vi "Begin.vi"() -> (0 "camera error out":errorcluster)   [LabVIEW 2013]
doc: "Called before other user functions, this VI is expected to open initial I/O refnums, load in file data, and do all program initialization. Notice that the <B>error out</B> terminal is simply used for data flow. Wiring it to other structures or subVIs ensures that this VI runs first."
uses:
  <vilib>/Rock Robotics/WPI/Encoder/WPI_EncoderType.ctl
  <vilib>/Rock Robotics/WPI/SafetyOutput/WPI_SafetyOutputConfigMenu.ctl
  <vilib>/Rock Robotics/WPI/DriverStation/WPI_DriverStationRobotMode2.ctl
  <vilib>/Rock Robotics/WPI/Joystick/WPI_JoystickDeviceEnum.ctl
  <vilib>/Rock Robotics/SystemInterfaces/DIO/FPGA_DIOPWMChannel.ctl
  <vilib>/Rock Robotics/WPI/Solenoid/WPI_SolenoidChannel.ctl
  <vilib>/Rock Robotics/SystemInterfaces/DIO/FPGA_DIOChannel.ctl
  <vilib>/Rock Robotics/WPI/Solenoid/WPI_SolenoidValue.ctl
  <vilib>/Rock Robotics/SystemInterfaces/AI/FPGA_AIChannel.ctl
  <vilib>/Rock Robotics/SystemInterfaces/AI/FPGA_AIGyroChannel.ctl
  <vilib>/Rock Robotics/WPI/Camera/WPI_CameraWhite Balance Values.ctl
  <vilib>/Rock Robotics/WPI/Camera/WPI_CameraExposure Values.ctl
  <vilib>/Rock Robotics/WPI/Camera/WPI_CameraFrameRate.ctl
  <vilib>/Rock Robotics/SystemInterfaces/DIO/FPGA_DIORelayChannel.ctl
  Robot Global Data.vi
  <vilib>/Rock Robotics/WPI/RobotDrive/WPI_RobotDriveOpen2MotorWithTalon.vi
  <vilib>/Rock Robotics/WPI/Solenoid/WPI_SolenoidOpenSingle.vi
  <vilib>/Rock Robotics/WPI/Counter/WPI_CounterDigitalInputToDigitalSource.vi
  <vilib>/Rock Robotics/WPI/Solenoid/WPI_SolenoidSetEnum.vi
  <vilib>/Rock Robotics/WPI/Counter/WPI_CounterOpen Gear Tooth Sensor Mode.vi
  <vilib>/Rock Robotics/WPI/RobotDrive/WPI_RobotDriveOpen4MotorWithTalon.vi
  <vilib>/Rock Robotics/WPI/Solenoid/WPI_SolenoidOpenDouble.vi
  <vilib>/Rock Robotics/WPI/Compressor/WPI_CompressorGetSetRefNum.vi
panel:
  in  "Number Samples to Average":u8=10 min=1 max=128
  in  "Decoding Type":T1=enum."4x"
  in  "DistancePerCount (deg)":dbl=0.11225
  in  "Minimum Rate":dbl=3.0
  in  "Gyro Gain (Volts/Degree/Second)":dbl=0.007
  # "Arm Encoder"
  # "0.13"
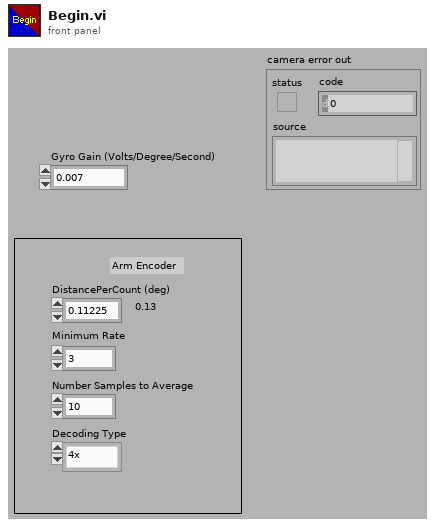
[diagram p1: front panel]
types:
  T1 = typedef "WPI_EncoderType.ctl" = enum16{"1x", "2x", "4x"}
  T2 = typedef "FPGA_DIORelayChannel.ctl" = enum8{"Relay 1", "Relay 2", "Relay 3", "Relay 4", "Relay 5", "Relay 6", "Relay 7", "Relay 8", "Invalid"}
  T3 = typedef "FPGA_DIOChannel.ctl" = enum8{"DIO 1", "DIO 2", "DIO 3", "DIO 4", "DIO 5", "DIO 6", "DIO 7", "DIO 8", "DIO 9", "DIO 10", "DIO 11", "DIO 12", "DIO 13", "DIO 14", "Invalid"}
  T4 = typedef "WPI_SolenoidChannel.ctl" = enum8{"Solenoid 1", "Solenoid 2", "Solenoid 3", "Solenoid 4", "Solenoid 5", "Solenoid 6", "Solenoid 7", "Solenoid 8", "Invalid"}
  T5 = typedef "WPI_CameraFrameRate.ctl" = u32
  T6 = typedef "WPI_CameraExposure Values.ctl" = enum16{"Auto", "Flicker-free 50 Hz", "Flicker-free 60 Hz", "Hold current"}
  T7 = typedef "WPI_CameraWhite Balance Values.ctl" = enum16{"Auto", "Fixed indoor", "Fixed outdoor 1", "Fixed outdoor 2", "Fixed fluorescent 1", "Fixed fluorescent 2", "Hold current"}
  T8 = typedef "FPGA_AIGyroChannel.ctl" = enum8{"AI 1", "AI 2", "Invalid"}
  T9 = typedef "FPGA_AIChannel.ctl" = enum8{"AI 1", "AI 2", "AI 3", "AI 4", "AI 5", "AI 6", "AI 7", "AI 8", "Invalid"}
  T10 = typedef "WPI_SolenoidValue.ctl" = enum16{"Off", "On", "Forward", "Reverse"}
  T11 = typedef "FPGA_DIOPWMChannel.ctl" = enum8{"PWM 1", "PWM 2", "PWM 3", "PWM 4", "PWM 5", "PWM 6", "PWM 7", "PWM 8", "PWM 9", "PWM 10", "Invalid"}
  T12 = typedef "WPI_JoystickDeviceEnum.ctl" = enum16{"USB 1", "USB 2", "USB 3", "USB 4", "Kinect 1", "Kinect 2"}
  T13 = typedef "WPI_DriverStationRobotMode2.ctl" = enum16{"Autonomous Disabled", "Autonomous Enabled", "Teleop Disabled", "Teleop Enabled", "Timeout", "Finish", "Test Disabled", "Test Enabled"}
  T14 = typedef "WPI_SafetyOutputConfigMenu.ctl" = enum16{"Enable", "Disable"}
  T15 = typedef "WPI_JoystickDevRef.ctl" = cluster{"Device":T12}
  T16 = typedef "WPI_DigitalInputDevRef.ctl" = cluster{"DevStatus":errorcluster, "DIO Channel":T3, "Digital Module":T17}
  T17 = typedef "FPGA_TypedefDigitalModule.ctl" = enum16{"Digital Module 1", "Digital Module 2"}
  T18 = typedef "FPGA_CounterEncoderSourceConvertionLVSourceType.ctl" = cluster{"DevStatus":errorcluster, "AnalogTriggerMode?":bool, "DigitalMode":cluster{"Digital Module":T17, "DIO Channel":T19}, "AnalogTriggerMode":cluster{"AnalogTriggerIndex":T20, "OutputType":T21}}
  T19 = typedef "FPGA_DIODigitalSourceChannel.ctl" = enum8{"DIO 1", "DIO 2", "DIO 3", "DIO 4", "DIO 5", "DIO 6", "DIO 7", "DIO 8", "DIO 9", "DIO 10", "DIO 11", "DIO 12", "DIO 13", "DIO 14", "Disabled"}
  T20 = typedef "FPGA_AnalogTriggerIndex.ctl" = enum8{"Trig 0", "Trig 1", "Trig 2", "Trig 3", "Trig 4", "Trig 5", "Trig 6", "Trig 7", "Invalid"}
  T21 = typedef "FPGA_AnalogTriggerOutType.ctl" = enum16{"InWindow", "TriggerState", "Rising", "Falling"}
  T22 = typedef "WPI_CounterDevRef.ctl" = cluster{"DevStatus":errorcluster, "CntIndex":T23}
  T23 = typedef "FPGA_CounterCtrSystemIndex.ctl" = enum8{"Ctr 0", "Ctr 1", "Ctr 2", "Ctr 3", "Ctr 4", "Ctr 5", "Ctr 6", "Ctr 7", "Invalid"}
  T24 = typedef "WPI_EncoderDevRef.ctl" = cluster{"DevStatus":errorcluster, "EncoderIndex":T25, "CounterIndex":T23, "DistancePerCount":dbl, "Decoding Type":T1}
  T25 = typedef "FPGA_EncoderIdx.ctl" = enum8{"Enc 0", "Enc 1", "Enc 2", "Enc 3", "Invalid"}
  T26 = typedef "WPI_CameraImageSize.ctl" = enum16{"640x480", "320x240", "160x120"}
  T27 = typedef "WPI_CameraDevRef.ctl" = cluster{"Camera Address":string, "CameraStatus":errorcluster, "Acquire Image Notifier":refnum<notifier>}
  T28 = typedef "WPI_RobotDriveDevRef.ctl" = cluster{"DevStatus":errorcluster, "Motors[]":T29[], "Square Inputs":bool, "Max Output":dbl, "Isochronous":bool}
  T29 = typedef "WPI_MotorControlDeviceRef.ctl" = cluster{"DeviceStatus":errorcluster, "Type":enum16{"PWM", "CAN"}, "PWM":cluster{"Digital Module":T17, "PWM Channel":T11, "DeadBand":T30}, "CAN":cluster{"Device Number":u8, "Control Mode":T31, "Semaphore":T32, "Max Vout":dbl}, "Invert":bool, "TransformRef":T33, "InvTransformRef":T33}
  T30 = typedef "WPI_PWMDeadband.ctl" = cluster{"Name":string, "maxPositivePwm":i32, "minPositivePwm":i32, "centerPwm":i32, "maxNegativePwm":i32, "minNegativePwm":i32, "angularRange":u16}
  T31 = typedef "WPI_CANJaguar_ControlMode.ctl" = enum8{"Percent VBus", "Current", "Speed", "Position", "Voltage"}
  T32 = typedef "Semaphore RefNum" = refnum<k1>
  T33 = typedef "WPI_PWMTransform_ConPane.ctl" = refnum<vi>
  T34 = typedef "WPI_GyroDevRef.ctl" = cluster{"DevStatus":errorcluster, "Analog Module":T35, "Analog Channel":T9, "Offset":dbl, "Gain (VoltsPerDegree/Second)":dbl}
  T35 = typedef "FPGA_TypedefAnalogModule.ctl" = enum16{"Analog Module 1", "Analog Module 2"}
  T36 = typedef "WPI_SolenoidDevRef.ctl" = cluster{"DevStatus":errorcluster, "Solenoid Module":T37, "Forward Solenoid Channel":T4, "Reverse Solenoid Channel":T4}
  T37 = typedef "FPGA_TypedefSolenoidModule.ctl" = enum16{"Solenoid Module 1", "Solenoid Module 2"}
  T38 = typedef "WPI_CompressorDevRef.ctl" = cluster{"DevStatus":errorcluster, "DigitalInputDevRef":T16, "RelayDevRef":T39}
  T39 = typedef "WPI_RelayDevRef.ctl" = cluster{"DevStatus":errorcluster, "Relay Channel":T2, "Digital Module":T17, "Relay Direction":T40}
  T40 = typedef "WPI_RelayDirection.ctl" = enum16{"Both directions", "Forward only", "Reverse only"}
  T41 = typedef "WPI_AnalogChannelDevRef.ctl" = cluster{"DevStatus":errorcluster, "Analog Module":T35, "Analog Channel":T9}
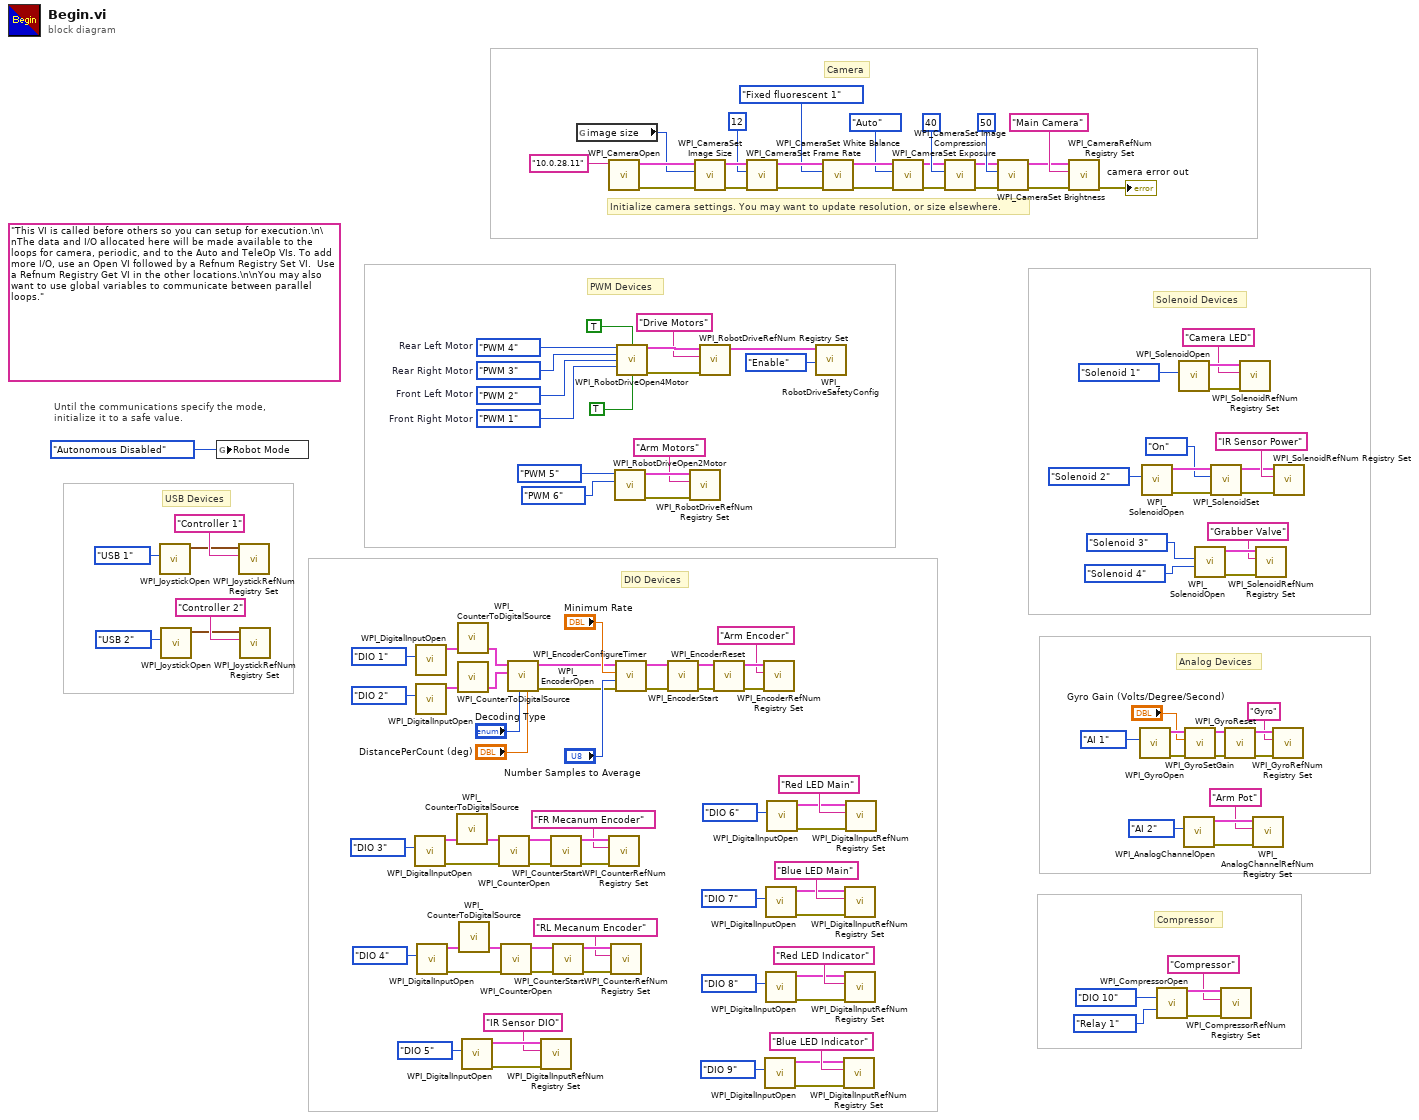
[diagram p0: block diagram]
diagram:
  w125 = FPGA_DIOPWMChannel."PWM 1"  # Front Right Motor
  w126 = FPGA_DIOPWMChannel."PWM 2"  # Front Left Motor
  w127 = FPGA_DIOPWMChannel."PWM 3"  # Rear Right Motor
  w128 = FPGA_DIOPWMChannel."PWM 4"  # Rear Left Motor
  (unwired) "This VI is called before others so you can setup for execution.\n\nThe data and I/O allocated here will be made available to the loops for camera, periodic, and to the Auto and TeleOp VIs. To add more I/O, use an Open VI followed by a Refnum Registry Set VI.  Use a Refnum Registry Get VI in the other locations.\n\nYou may also want to use global variables to communicate between parallel loops."
  # "Compressor"
  # "Camera"
  # "Initialize camera settings. You may want to update resolution, or size elsewhere."
  # "Analog Devices"
  # "DIO Devices"
  # "Solenoid Devices"
  # "USB Devices"
  # "PWM Devices"
  # "Until the communications specify the mode,\ninitialize it to a safe value."
  n1 = call <vilib>:"WPI_JoystickOpen.vi"("JoystickDevice"=WPI_JoystickDeviceEnum."USB 1") -> ("JoystickDevRef"=w130:T15)  [unwired: 10 in]
  n2 = call <vilib>:"WPI_JoystickOpen.vi"("JoystickDevice"=WPI_JoystickDeviceEnum."USB 2") -> ("JoystickDevRef"=w123:T15)  [unwired: 10 in]
  n3 = global write "Robot Global Data.vi" "Robot Mode"(WPI_DriverStationRobotMode2."Autonomous Disabled" ("Robot Mode")) -> ()
  n4 = call <vilib>:"WPI_JoystickRefNum Registry Set.vi"("refnum name"="Controller 1", "JoystickDevRef"=w130) -> ()  [unwired: 8 in, 2 out]
  n5 = call <vilib>:"WPI_JoystickRefNum Registry Set.vi"("refnum name"="Controller 2", "JoystickDevRef"=w123) -> ()  [unwired: 8 in, 2 out]
  n6 = call <vilib>:"WPI_DigitalInputOpen.vi"("DIO Channel"=FPGA_DIOChannel."DIO 3") -> ("error out"=w82:errorcluster, "DigitalInputDevRef"=w101:T16)  [unwired: 9 in]
  n7 = call <vilib>:"WPI_DigitalInputOpen.vi"("DIO Channel"=FPGA_DIOChannel."DIO 1") -> ("DigitalInputDevRef"=w113:T16)  [unwired: 9 in, 1 out]
  n8 = call <vilib>:"WPI_DigitalInputOpen.vi"("DIO Channel"=FPGA_DIOChannel."DIO 2") -> ("DigitalInputDevRef"=w110:T16)  [unwired: 9 in, 1 out]
  n9 = call <vilib>:"WPI_DigitalInputOpen.vi"("DIO Channel"=FPGA_DIOChannel."DIO 4") -> ("error out"=w83:errorcluster, "DigitalInputDevRef"=w93:T16)  [unwired: 9 in]
  n10 = call-poly <vilib>:"WPI_CounterToDigitalSource.vi"("DigitalInputDevRef"=w101) -> ("Digital Source"=w99:T18)  [unwired: 6 in]
  n11 = call-poly <vilib>:"WPI_CounterToDigitalSource.vi"("DigitalInputDevRef"=w113) -> ("Digital Source"=w21:T18)  [unwired: 6 in]
  n12 = call-poly <vilib>:"WPI_CounterToDigitalSource.vi"("DigitalInputDevRef"=w110) -> ("Digital Source"=w20:T18)  [unwired: 6 in]
  n13 = call-poly <vilib>:"WPI_CounterToDigitalSource.vi"("DigitalInputDevRef"=w93) -> ("Digital Source"=w91:T18)  [unwired: 6 in]
  n14 = call <vilib>:"WPI_DigitalInputOpen.vi"("DIO Channel"=FPGA_DIOChannel."DIO 5") -> ("error out"=w84:errorcluster, "DigitalInputDevRef"=w85:T16)  [unwired: 9 in]
  n15 = call-poly <vilib>:"WPI_CounterOpen.vi"("error in (no error)"=w82, "Source"=w99) -> ("error out"=w98:errorcluster, "CounterDevRef"=w97:T22)  [unwired: 8 in]
  n16 = call-poly <vilib>:"WPI_CounterOpen.vi"("error in (no error)"=w83, "Source"=w91) -> ("error out"=w90:errorcluster, "CounterDevRef"=w89:T22)  [unwired: 8 in]
  n17 = call <vilib>:"WPI_EncoderOpen.vi"("DistancePerCount"="DistancePerCount (deg)", "Decoding Type"="Decoding Type", "BSource"=w20, "ASource"=w21) -> ("error out"=w14:errorcluster, "EncoderDevRef"=w15:T24)  [unwired: 4 in, 2 out]
  n18 = call <vilib>:"WPI_DigitalInputRefNum Registry Set.vi"("error in (no error)"=w84, "refnum name"="IR Sensor DIO", "DigitalInputDevRef"=w85) -> ()  [unwired: 7 in, 2 out]
  n19 = call <vilib>:"WPI_CounterStart.vi"("error in (no error)"=w98, "CounterDevRef in"=w97) -> ("error out"=w96:errorcluster, "CounterDevRef out"=w95:T22)  [unwired: 8 in]
  n20 = call <vilib>:"WPI_CounterStart.vi"("error in (no error)"=w90, "CounterDevRef in"=w89) -> ("error out"=w88:errorcluster, "CounterDevRef out"=w87:T22)  [unwired: 8 in]
  n21 = global read "Robot Global Data.vi" "image size"() -> (w43:T26)
  n22 = call <vilib>:"WPI_CameraOpen.vi"("Camera Address"="10.0.28.11") -> ("error out"=w55:errorcluster, "CameraDevRef"=w56:T27)  [unwired: 1 in, 8 out]
  n23 = call <vilib>:"WPI_CounterRefNum Registry Set.vi"("error in (no error)"=w96, "refnum name"="FR Mecanum Encoder", "CounterDevRef"=w95) -> ()  [unwired: 7 in, 2 out]
  n24 = call <vilib>:"WPI_CounterRefNum Registry Set.vi"("error in (no error)"=w88, "refnum name"="RL Mecanum Encoder", "CounterDevRef"=w87) -> ()  [unwired: 7 in, 2 out]
  n25 = call-poly <vilib>:"WPI_RobotDriveOpen2Motor.vi"("Right Motor"=FPGA_DIOPWMChannel."PWM 6", "Left Motor"=FPGA_DIOPWMChannel."PWM 5") -> ("error out"=w118:errorcluster, "RobotDriveDevRef"=w119:T28)  [unwired: 8 in]
  n26 = call <vilib>:"WPI_EncoderConfigureTimer.vi"("error in (no error)"=w14, "Number Samples to Average"="Number Samples to Average", "Minimum Rate"="Minimum Rate", "EncoderDevRef"=w15) -> ("error out"=w11:errorcluster, "EncoderDevRef"=w12:T24)  [unwired: 6 out]
  n27 = call-poly <vilib>:"WPI_RobotDriveOpen4Motor.vi"("Rear Left Motor"=w128, "Rear Right Motor Inverted"=TRUE, "Rear Right Motor"=w127, "Front Left Motor"=w126, "Front Right Motor"=w125, "Front Right Motor Inverted"=TRUE) -> ("RobotDriveDevRef"=w137:T28, "error out"=w135:errorcluster)  [unwired: 8 in]
  n28 = call <vilib>:"WPI_EncoderStart.vi"("error in (no error)"=w11, "EncoderDevRef"=w12) -> ("error out"=w10:errorcluster, "EncoderDevRef"=w13:T24)  [unwired: 8 out]
  n29 = call <vilib>:"WPI_RobotDriveRefNum Registry Set.vi"("error in (no error)"=w118, "refnum name"="Arm Motors", "RobotDriveDevRef"=w119) -> ()  [unwired: 7 in, 2 out]
  n30 = call <vilib>:"WPI_CameraSet Image Size.vi"("error in (no error)"=w55, "Image Size"=w43, "CameraDevRef"=w56) -> ("error out"=w54:errorcluster, "CameraDevRef Out"=w57:T27)  [unwired: 7 out]
  n31 = call <vilib>:"WPI_RobotDriveRefNum Registry Set.vi"("error in (no error)"=w135, "refnum name"="Drive Motors", "RobotDriveDevRef"=w137) -> ("RobotDriveDevRef"=w134:T28)  [unwired: 8 out]
  n32 = call <vilib>:"WPI_EncoderReset.vi"("error in (no error)"=w10, "EncoderDevRef"=w13) -> ("error out"=w9:errorcluster, "EncoderDevRef"=w8:T24)  [unwired: 8 out]
  n33 = call <vilib>:"WPI_CameraSet Frame Rate.vi"("error in (no error)"=w54, "Frame Rate (fps)"=T5 12, "CameraDevRef"=w57) -> ("error out"=w53:errorcluster, "CameraDevRef Out"=w59:T27)  [unwired: 7 out]
  n34 = call <vilib>:"WPI_EncoderRefNum Registry Set.vi"("error in (no error)"=w9, "refnum name"="Arm Encoder", "EncoderDevRef"=w8) -> ()  [unwired: 7 in, 2 out]
  n35 = call <vilib>:"WPI_DigitalInputOpen.vi"("DIO Channel"=FPGA_DIOChannel."DIO 9") -> ("error out"=w29:errorcluster, "DigitalInputDevRef"=w26:T16)  [unwired: 9 in]
  n36 = call <vilib>:"WPI_DigitalInputOpen.vi"("DIO Channel"=FPGA_DIOChannel."DIO 7") -> ("error out"=w37:errorcluster, "DigitalInputDevRef"=w34:T16)  [unwired: 9 in]
  n37 = call <vilib>:"WPI_DigitalInputOpen.vi"("DIO Channel"=FPGA_DIOChannel."DIO 8") -> ("error out"=w33:errorcluster, "DigitalInputDevRef"=w30:T16)  [unwired: 9 in]
  n38 = call <vilib>:"WPI_DigitalInputOpen.vi"("DIO Channel"=FPGA_DIOChannel."DIO 6") -> ("error out"=w41:errorcluster, "DigitalInputDevRef"=w38:T16)  [unwired: 9 in]
  n39 = call <vilib>:"WPI_RobotDriveSafetyConfig.vi"("mode"=WPI_SafetyOutputConfigMenu."Enable", "RobotDriveDevRef"=w134) -> ()  [unwired: 8 in, 2 out]
  n40 = call <vilib>:"WPI_CameraSet White Balance.vi"("error in (no error)"=w53, "White Balance"=WPI_CameraWhite_Balance_Values."Fixed fluorescent 1", "CameraDevRef"=w59) -> ("error out"=w52:errorcluster, "CameraDevRef Out"=w58:T27)  [unwired: 7 out]
  n41 = call <vilib>:"WPI_DigitalInputRefNum Registry Set.vi"("error in (no error)"=w29, "refnum name"="Blue LED Indicator", "DigitalInputDevRef"=w26) -> ()  [unwired: 7 in, 2 out]
  n42 = call <vilib>:"WPI_DigitalInputRefNum Registry Set.vi"("error in (no error)"=w37, "refnum name"="Blue LED Main", "DigitalInputDevRef"=w34) -> ()  [unwired: 7 in, 2 out]
  n43 = call <vilib>:"WPI_DigitalInputRefNum Registry Set.vi"("error in (no error)"=w33, "refnum name"="Red LED Indicator", "DigitalInputDevRef"=w30) -> ()  [unwired: 7 in, 2 out]
  n44 = call <vilib>:"WPI_DigitalInputRefNum Registry Set.vi"("error in (no error)"=w41, "refnum name"="Red LED Main", "DigitalInputDevRef"=w38) -> ()  [unwired: 7 in, 2 out]
  n45 = call <vilib>:"WPI_CameraSet Exposure.vi"("error in (no error)"=w52, "Exposure"=WPI_CameraExposure_Values."Auto", "CameraDevRef"=w58) -> ("error out"=w51:errorcluster, "CameraDevRef Out"=w61:T27)  [unwired: 7 out]
  n46 = call <vilib>:"WPI_CameraSet Image Compression.vi"("error in (no error)"=w51, "Compression"=40, "CameraDevRef"=w61) -> ("error out"=w50:errorcluster, "CameraDevRef Out"=w60:T27)  [unwired: 7 out]
  n47 = call <vilib>:"WPI_CameraSet Brightness.vi"("error in (no error)"=w50, "Brightness"=50, "CameraDevRef"=w60) -> ("error out"=w48:errorcluster, "CameraDevRef Out"=w49:T27)  [unwired: 7 out]
  n48 = call <vilib>:"WPI_CameraRefNum Registry Set.vi"("error in (no error)"=w48, "refnum name"="Main Camera", "CameraDevRef"=w49) -> ("error out"=→"camera error out":errorcluster)  [unwired: 8 out]
  n49 = call <vilib>:"WPI_GyroOpen.vi"("Analog Channel"=FPGA_AIGyroChannel."AI 1") -> ("error out"=w71:errorcluster, "GyroDevRef"=w73:T34)  [unwired: 5 in, 4 out]
  n50 = call-poly <vilib>:"WPI_SolenoidOpen.vi"("Solenoid Channel"=WPI_SolenoidChannel."Solenoid 2") -> ("error out"=w104:errorcluster, "SolenoidDevRef"=w103:T36)  [unwired: 9 in]
  n51 = call <vilib>:"WPI_CompressorOpen.vi"("Pressure Switch DIO Channel"=FPGA_DIOChannel."DIO 10", "Relay Channel"=FPGA_DIORelayChannel."Relay 1") -> ("CompressorDevRef"=w5:T38, "error out"=w6:errorcluster)  [unwired: 12 in]
  n52 = call-poly <vilib>:"WPI_SolenoidOpen.vi"("Solenoid Channel"=WPI_SolenoidChannel."Solenoid 1") -> ("error out"=w111:errorcluster, "SolenoidDevRef"=w115:T36)  [unwired: 9 in]
  n53 = call <vilib>:"WPI_AnalogChannelOpen.vi"("Analog Channel"=FPGA_AIChannel."AI 2") -> ("error out"=w78:errorcluster, "AIDeviceRef"=w77:T41)  [unwired: 9 in]
  n54 = call <vilib>:"WPI_GyroSetGain.vi"("error in (no error)"=w71, "Gain (VoltsPerDegree/Second)"="Gyro Gain (Volts/Degree/Second)", "GyroDevRef"=w73) -> ("error out"=w75:errorcluster, "GyroDevRef"=w74:T34)  [unwired: 7 out]
  n55 = call-poly <vilib>:"WPI_SolenoidOpen.vi"("Reverse Solenoid Channel"=WPI_SolenoidChannel."Solenoid 4" ("Solenoid Channel"), "Forward Solenoid Channel"=WPI_SolenoidChannel."Solenoid 3" ("Solenoid Channel")) -> ("error out"=w22:errorcluster, "SolenoidDevRef"=w24:T36)  [unwired: 8 in]
  n56 = call-poly <vilib>:"WPI_SolenoidSet.vi"("error in (no error)"=w104, "Value"=WPI_SolenoidValue."On", "SolenoidDevRef"=w103) -> ("error out"=w105:errorcluster, "SolenoidDevRef"=w106:T36)  [unwired: 7 in]
  n57 = call <vilib>:"WPI_CompressorRefNum Registry Set.vi"("error in (no error)"=w6, "refnum name"="Compressor", "CompressorDevRef"=w5) -> ()  [unwired: 7 in, 2 out]
  n58 = call <vilib>:"WPI_GyroReset.vi"("error in (no error)"=w75, "GyroDevRef"=w74) -> ("error out"=w69:errorcluster, "GyroDevRef"=w68:T34)  [unwired: 8 out]
  n59 = call <vilib>:"WPI_SolenoidRefNum Registry Set.vi"("error in (no error)"=w111, "refnum name"="Camera LED", "SolenoidDevRef"=w115) -> ()  [unwired: 7 in, 2 out]
  n60 = call <vilib>:"WPI_AnalogChannelRefNum Registry Set.vi"("error in (no error)"=w78, "refnum name"="Arm Pot", "AIDeviceRef"=w77) -> ()  [unwired: 7 in, 2 out]
  n61 = call <vilib>:"WPI_SolenoidRefNum Registry Set.vi"("error in (no error)"=w22, "refnum name"="Grabber Valve", "SolenoidDevRef"=w24) -> ()  [unwired: 7 in, 2 out]
  n62 = call <vilib>:"WPI_GyroRefNum Registry Set.vi"("error in (no error)"=w69, "refnum name"="Gyro", "GyroDevRef"=w68) -> ()  [unwired: 7 in, 2 out]
  n63 = call <vilib>:"WPI_SolenoidRefNum Registry Set.vi"("error in (no error)"=w105, "refnum name"="IR Sensor Power", "SolenoidDevRef"=w106) -> ()  [unwired: 7 in, 2 out]
